vi "GetGitHash.vi"(11 "git hash file path":path=path "C:/Users/jmckenna/MIDAS_GEM_LabVIEW/.git/HEAD/refs/heads/master\n") -> (2 "git hash (version)":string, 3 "Branch":string)   [LabVIEW 2018]
uses:
  <userlib>/_RADE/MTA-lib/file/file.llb/Valid Path - Traditional__ogtk.vi
  <userlib>/_RADE/MTA-lib/file/file.llb/Strip Path - Traditional__ogtk.vi
panel:
  out "error out":errorcluster
  out "stripped path":path
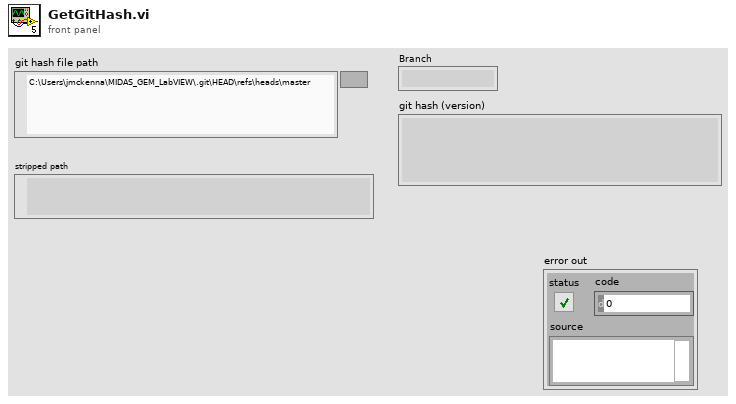
[diagram p1: front panel]
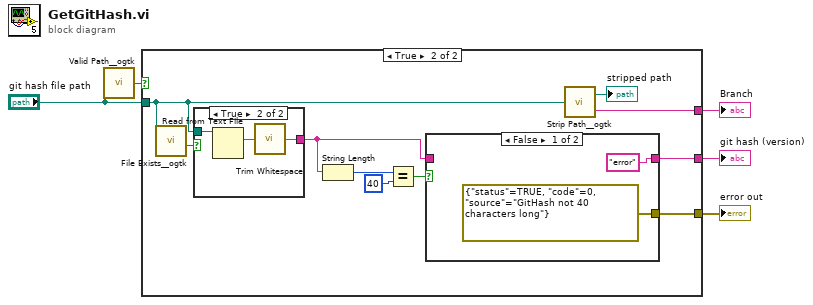
[diagram p0: block diagram]
diagram:
  n1 = call-poly <userlib>:"Valid Path__ogtk.vi"("path"="git hash file path") -> ("valid"=w5:bool)
  n2 = case shown="True" w5 {
    tunnel: "git hash file path" -> [_ w13]
    tunnel: [_ w11] -> w3
    tunnel: [_ w12] -> w2
    tunnel: [_ w6] -> w1
    frame False {
    }
    frame True {
      n3 = call <userlib>:"File Exists__ogtk.vi"("file path"=w13) -> ("exists"=w15:bool)  [unwired: 6 in, 1 out]
      n4 = case shown="True" w15 {
        tunnel: w13 -> [_ w21]
        tunnel: [_ w19] -> w10
        frame False {
        }
        frame True {
          n5 = Read from Text File(file (use dialog)=w21) -> (text=w20:string)  [unwired: 3 in, 3 out]
          n6 = call <vilib>:"Trim Whitespace.vi"("string"=w20) -> ("trimmed string"=w19:string)  [unwired: 1 in]
        }
      }
      n7 = String Length(string=w10) -> (length=w9:i32)
      n8 = Equal?(x=w9, y=40) -> (x = y?=w7:bool)
      n9 = case shown="False" w7 {
        tunnel: ["error" ("trimmed string") w18] -> w11
        tunnel: w10 -> [_ w18]
        tunnel: [errorcluster {"status"=TRUE, "code"=0, "source"="GitHash not 40 characters long"} ("error out") _] -> w6
        frame False {
        }
        frame True {
        }
      }
      n10 = call-poly <userlib>:"Strip Path__ogtk.vi"("path"=w13) -> ("stripped path"=→"stripped path":path, "name"=w12:string)
    }
  }
  "git hash (version)" <- w3
  "Branch" <- w2
  "error out" <- w1
